vi "PostRunCTRL.vi"(8 "error in (no error)":errorcluster) -> (0 "error out":errorcluster)   [LabVIEW 2017, in "programControl.lvlib"]
doc: "This VI releases the program control module Queue and User Event"
uses:
  programControl.lvlib
  Queue/TypeDefs/queueFGVState.ctl
  StartUEFGV/TypeDefs/UEFGVcontrol.ctl
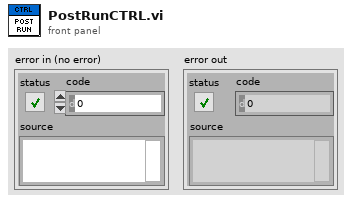
[diagram p1: front panel]
types:
  T1 = typedef "UEFGVcontrol.ctl" = enum16{"Create", "Get", "Destroy"}
  T2 = typedef "programControl.lvlib/queueFGVState.ctl" = enum16{"obtain", "enqueue (low priority)", "enqueue (high priority)", "dequeue", "release"}
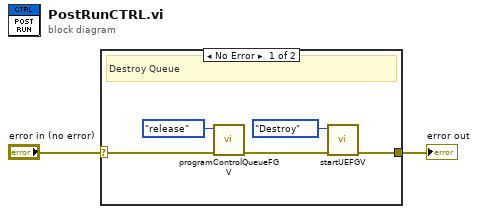
[diagram p0: block diagram]
diagram:
  n1 = case shown="No Error" "error in (no error)" {
    selector: "error in (no error)" -> [w7 w8]
    tunnel: [w4 w8] -> w1
    frame No Error {
      # "Destroy Queue"
      n2 = call "programControlQueueFGV.vi"("error in (no error)"=w7, "Enum"=queueFGVState."release") -> ("error out"=w5:errorcluster)  [unwired: 8 in, 1 out]
      n3 = call "startUEFGV.vi"("error in (no error)"=w5, "Enum"=UEFGVcontrol."Destroy") -> ("error out"=w4:errorcluster)  [unwired: 8 in, 1 out]
    }
    frame Error {
    }
  }
  "error out" <- w1
